vi "计算两条直线的交点（斜率与截距）.vi"(8 "Error In":errorcluster caption="错误输入", 10 "直线B":T1, 11 "直线A":T1) -> (0 "Error Out":errorcluster caption="错误输出", 3 "交点":T2)   [LabVIEW 2012, in "几何工具.lvlib"]
uses:
  <vilib>/Utility/miscctls.llb/LVPointDoubleTypeDef.ctl
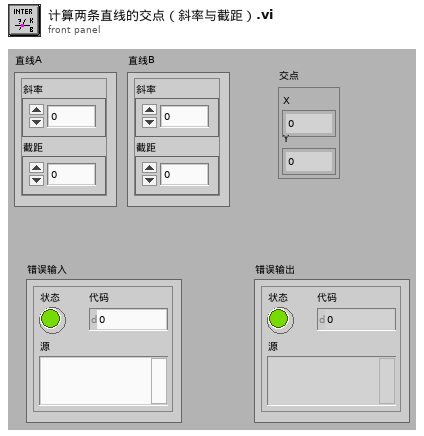
[diagram p1: front panel]
types:
  T1 = typedef "几何工具.lvlib/斜率与截距.ctl" = cluster{"斜率":dbl, "截距":dbl}
  T2 = typedef "LVPointDoubleTypeDef.ctl" = cluster{"X":dbl, "Y":dbl}
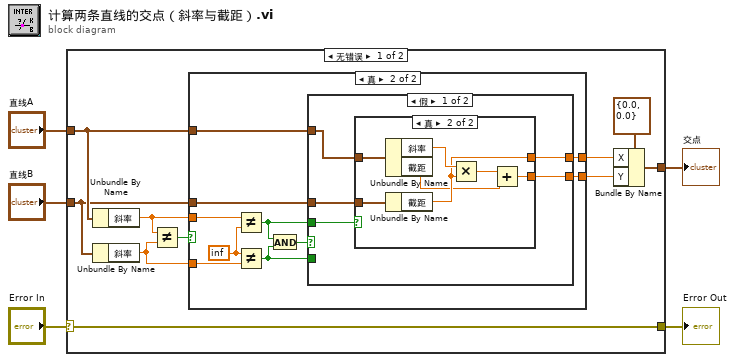
[diagram p0: block diagram]
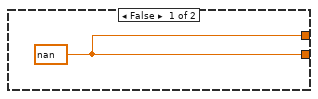
[diagram p2: hidden frame]
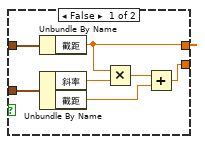
[diagram p3: hidden frame]
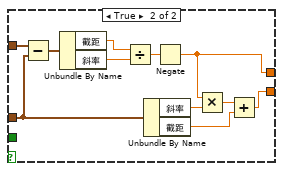
[diagram p4: hidden frame]
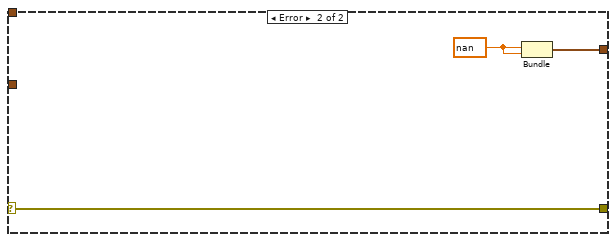
[diagram p5: hidden frame]
diagram:
  n1 = case shown="无错误" "Error In" {
    selector: "Error In" -> [w15 w59]
    tunnel: [w15 w59] -> w4
    tunnel: "直线A" -> [w11 _]
    tunnel: "直线B" -> [w10 _]
    tunnel: [w12 w57] -> w1
    frame No Error {
      n2 = Unbundle By Name(w11) -> ("斜率"=w7:dbl)
      n3 = Unbundle By Name(w10) -> ("斜率"=w6:dbl)
      n4 = Not Equal?(x=w7, y=w6) -> (x != y?=w8:bool)
      n5 = case shown="真" w8 {
        tunnel: [w16 w26] -> w14
        tunnel: [w16 w25] -> w13
        tunnel: w11 -> [_ w24]
        tunnel: w10 -> [_ w23]
        tunnel: w7 -> [_ w22]
        tunnel: w6 -> [_ w20]
        frame False {
          w16 = nan
        }
        frame True {
          w21 = inf
          n6 = Not Equal?(x=w22, y=w21) -> (x != y?=w18:bool)
          n7 = Not Equal?(x=w21, y=w20) -> (x != y?=w17:bool)
          n8 = And(x=w18, y=w17) -> (x .and. y?=w19:bool)
          n9 = case shown="假" w19 {
            tunnel: [w27 w56] -> w26
            tunnel: [w28 w53] -> w25
            tunnel: w24 -> [w30 w47]
            tunnel: w23 -> [w29 w46]
            tunnel: w18 -> [w31 _]
            tunnel: w17 -> [_ _]
            frame False {
              n10 = case shown="真" w31 {
                tunnel: w30 -> [w37 w45]
                tunnel: w29 -> [w38 w44]
                tunnel: [w36 w42] -> w28
                tunnel: [w32 w39] -> w27
                frame False {
                  n11 = Unbundle By Name(w37) -> ("截距"=w36:dbl)
                  n12 = Unbundle By Name(w38) -> ("斜率"=w35:dbl, "截距"=w33:dbl)
                  n13 = Multiply(x=w36, y=w35) -> (x*y=w34:dbl)
                  n14 = Add(x=w34, y=w33) -> (x+y=w32:dbl)
                }
                frame True {
                  n15 = Unbundle By Name(w45) -> ("斜率"=w43:dbl, "截距"=w40:dbl)
                  n16 = Unbundle By Name(w44) -> ("截距"=w42:dbl)
                  n17 = Multiply(x=w43, y=w42) -> (x*y=w41:dbl)
                  n18 = Add(x=w41, y=w40) -> (x+y=w39:dbl)
                }
              }
            }
            frame True {
              n19 = Subtract(x=w47, y=w46) -> (x-y=w48:T1)
              n20 = Unbundle By Name(w48) -> ("截距"=w49:dbl, "斜率"=w50:dbl)
              n21 = Divide(x=w49, y=w50) -> (x/y=w51:dbl)
              n22 = Unbundle By Name(w46) -> ("斜率"=w52:dbl, "截距"=w55:dbl)
              n23 = Negate(x=w51) -> (-x=w53:dbl)
              n24 = Multiply(x=w53, y=w52) -> (x*y=w54:dbl)
              n25 = Add(x=w54, y=w55) -> (x+y=w56:dbl)
            }
          }
        }
      }
      n26 = Bundle By Name(cluster=T2 {"X"=0.0, "Y"=0.0} ("Double Point"), "X"=w13, "Y"=w14) -> (w12:T2)
    }
    frame Error {
      w58 = nan
      n27 = Bundle(w58, w58) -> (w57:cluster{dbl, dbl})  [unwired: 1 in]
    }
  }
  "Error Out" <- w4
  "交点" <- w1
